vi "ETH_1 Main.vi"(8 "error in":errorcluster, 10 "data in":string, 11 "ETH1-Q":refnum<queue>) -> (0 "error out":errorcluster)   [LabVIEW 2022 SP3]
panel:
  out "overflow?":bool
  out "Motor FB LR":u32
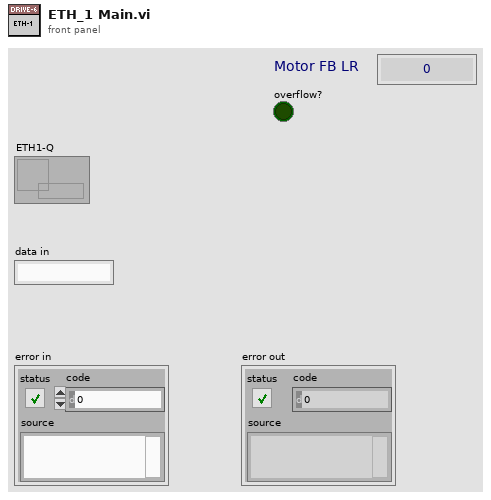
[diagram p1: front panel]
types:
  T1 = cluster{"Run ACK":dbl, "Frequency":dbl, "Speed":dbl, "RPM Dir":dbl, "VDC":dbl, "IDC":dbl, "Movable IDC":dbl, "M-State":dbl}
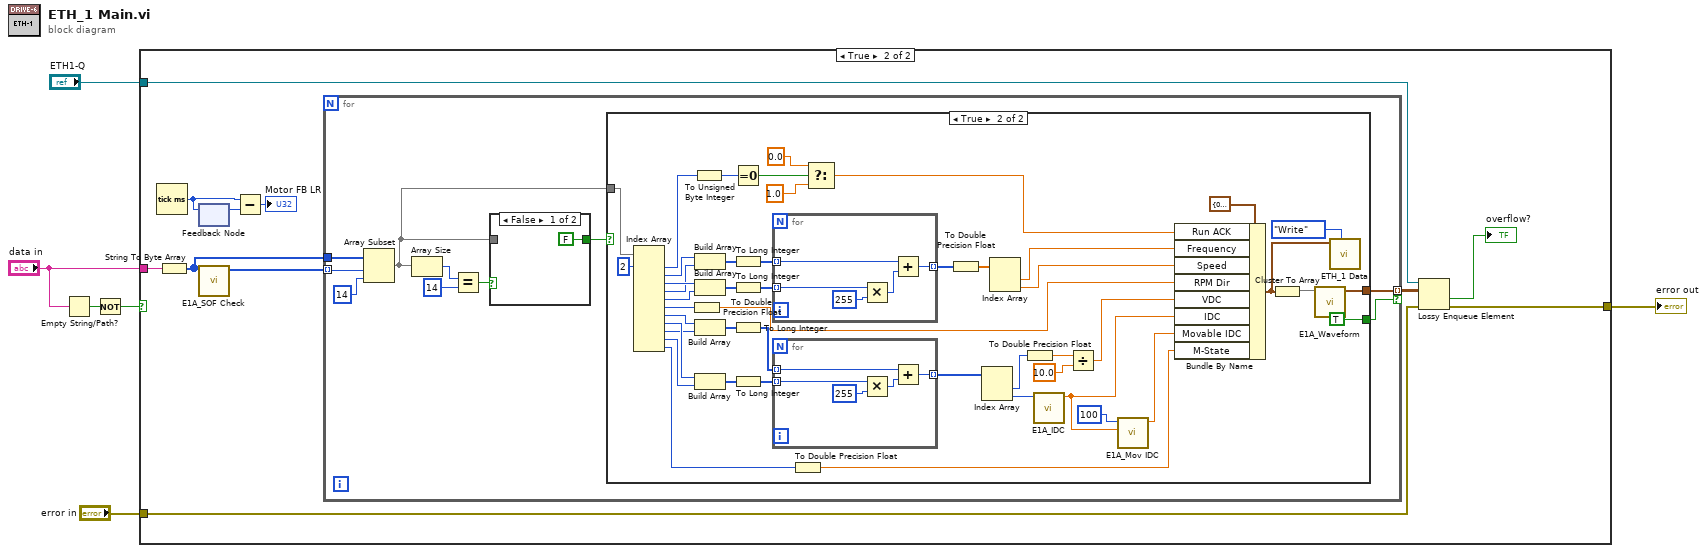
[diagram p0: block diagram]
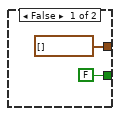
[diagram p3: hidden frame]
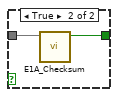
[diagram p4: hidden frame]
diagram:
  n1 = Empty String/Path?(string/path="data in") -> (empty?=w6:bool)
  n2 = Not(x=w6) -> (.not. x?=w5:bool)
  n3 = case shown="True" w5 {
    tunnel: "data in" -> [_ w18]
    tunnel: "ETH1-Q" -> [_ w14]
    tunnel: "error in" -> [w7 w13]
    tunnel: [w7 w12] -> w1
    frame False {
    }
    frame True {
      n4 = Tick Count (ms)() -> (millisecond timer value=w11:u32)
      n5 = String To Byte Array(string=w18) -> (unsigned byte array=w16:u8[])
      n6 = feedback #1() -> (w10:u32)  [unwired: 1 in]
      n7 = feedback-in #1(w11) -> ()
      n8 = call "E1A_SOF Check.vi"("Bytes data in"=w16) -> ("index of passed smpl"=w17:i32[])  [unwired: 8 in, 2 out]
      n9 = Subtract(x=w11, y=w10) -> (x-y=→"Motor FB LR":u32)
      n10 = for {
        tunnel: w17 -> [w25] mode=indexing
        tunnel: w16 -> [w24]
        tunnel: [w20] -> w15 mode=indexing if=w19
        n11 = Array Subset(array=w24, index=w25, length=14) -> (w21:u8[])
        n12 = Array Size(array=w21) -> (size(s)=w27:i32)
        n13 = Equal?(x=w27, y=14) -> (x = y?=w23:bool)
        n14 = case shown="False" w23 {
          tunnel: w21 -> [_ w90]
          tunnel: [FALSE ("Checksum") w89] -> w22
          frame False {
          }
          frame True {
            n15 = call "E1A_Checksum.vi"("Data"=w90) -> ("Checksum"=w89:bool)  [unwired: 10 in]
          }
        }
        n16 = case shown="True" w22 {
          tunnel: w21 -> [_ w53]
          tunnel: [waveform(dbl)[] [] ("WF out") w34] -> w20
          tunnel: [FALSE TRUE] -> w19
          frame False {
          }
          frame True {
            n17 = Index Array(array=w53, index #1=2 ("index")) -> (element #1=w75:u8, element #2=w69:u8, element #3=w68:u8, element #4=w67:u8, element #5=w66:u8, element #6=w64:u8, element #7=w59:u8, element #8=w58:u8, element #9=w57:u8, element #10=w56:u8, element #11=w52:u8)  [unwired: 10 in]
            n18 = To Double Precision Float(number=w64) -> (double precision float=w43:dbl)
            n19 = To Unsigned Byte Integer(number=w75) -> (unsigned 8bit integer=w76:u8)
            n20 = Build Array(w69, w67) -> (w74:u8[])
            n21 = Build Array(w68, w66) -> (w73:u8[])
            n22 = Build Array(w59, w57) -> (w63:u8[])
            n23 = Build Array(w58, w56) -> (w62:u8[])
            n24 = Equal To 0?(x=w76) -> (x = 0?=w77:bool)
            n25 = To Long Integer(number=w74) -> (32bit integer=w71:i32[])
            n26 = To Long Integer(number=w73) -> (32bit integer=w70:i32[])
            n27 = To Long Integer(number=w63) -> (32bit integer=w61:i32[])
            n28 = To Long Integer(number=w62) -> (32bit integer=w60:i32[])
            n29 = for {
              tunnel: w71 -> [w87] mode=indexing
              tunnel: w70 -> [w86] mode=indexing
              tunnel: [w84] -> w72 mode=indexing
              n30 = Multiply(x=w86, y=255) -> (x*y=w85:i32)
              n31 = Add(x=w87, y=w85) -> (x+y=w84:i32)
            }
            n32 = for {
              tunnel: w61 -> [w82] mode=indexing
              tunnel: w60 -> [w81] mode=indexing
              tunnel: [w79] -> w41 mode=indexing
              n33 = Multiply(x=w81, y=255) -> (x*y=w80:i32)
              n34 = Add(x=w82, y=w80) -> (x+y=w79:i32)
            }
            n35 = To Double Precision Float(number=w52) -> (double precision float=w36:dbl)
            n36 = Select(t=0.0, s=w77, f=1.0) -> (s? t:f=w49:dbl)
            n37 = To Double Precision Float(number=w72) -> (double precision float=w65:dbl[])
            n38 = Index Array(array=w41) -> (element #1=w45:i32, element #2=w40:i32)  [unwired: 2 in]
            n39 = Index Array(array=w65) -> (element #1=w48:dbl, element #2=w44:dbl)  [unwired: 2 in]
            n40 = To Double Precision Float(number=w45) -> (double precision float=w47:dbl)
            n41 = call "E1A_IDC.vi"("IDC in"=w40) -> ("IDC out"=w39:dbl)  [unwired: 10 in]
            n42 = Divide(x=w47, y=10.0) -> (x/y=w42:dbl)
            n43 = call "E1A_Mov IDC.vi"("Idc"=w39, "SampleSize"=100) -> ("Mean"=w37:dbl)  [unwired: 9 in]
            n44 = Bundle By Name(cluster=T1 {"Run ACK"=0.0, "Frequency"=0.0, "Speed"=0.0, "RPM Dir"=0.0, "VDC"=0.0, "IDC"=0.0, "Movable IDC"=0.0, "M-State"=0.0} ("output cluster"), "Run ACK"=w49, "Frequency"=w48, "Speed"=w44, "RPM Dir"=w43, "VDC"=w42, "IDC"=w39, "Movable IDC"=w37, "M-State"=w36) -> (w31:T1)
            n45 = Cluster To Array(cluster=w31) -> (array=w35:dbl[])
            n46 = call "E1A_Waveform.vi"("Data in"=w35) -> ("WF out"=w34:waveform(dbl)[])  [unwired: 10 in]
            n47 = call "ETH_1 Data.vi"("Enum"=enum16{"Read", "Write"}."Write", "ETH_1"=w31) -> ()  [unwired: 8 in, 2 out]
          }
        }
      }
      n48 = Lossy Enqueue Element(queue=w14, element=w15, error in (no error)=w13) -> (overflow?=→"overflow?":bool, error out=w12:errorcluster)  [unwired: 2 out]
    }
  }
  "error out" <- w1
